vi "map Modbus channels.vi"(8 "error in":errorcluster, 10 "mapping":T1, 11 "Modbus Slave configuration in":refnum<class "Modbus Module configuration.lvclass">) -> (0 "error out":errorcluster, 3 "Modbus Slave configuration out":refnum<class "Modbus Module configuration.lvclass">)   [LabVIEW 2013, in "Modbus Module configuration.lvclass"]
uses:
  Modbus Module configuration.lvclass
  modbus mapping behavior.ctl
  Modbus Module configuration.lvclass/Modbus Module configuration.ctl
  <vilib>/NI/Tag Bus Module Framework/channel/channel classification.ctl
  module channel/data bank type.ctl
  <vilib>/NI/Tag Bus Module Framework/channel/TBM channel.lvclass/TBM channel.ctl
  module channel/Modbus Module Channel.lvclass/Modbus Module Channel.ctl
  <vilib>/NI/Tag Bus Module Framework/channel/Read channel classification.vi
  module channel/Read modbus type.vi
  module channel/Modbus Module Channel.lvclass
  <vilib>/NI/Tag Bus Module Framework/channel/TBM channel.lvclass
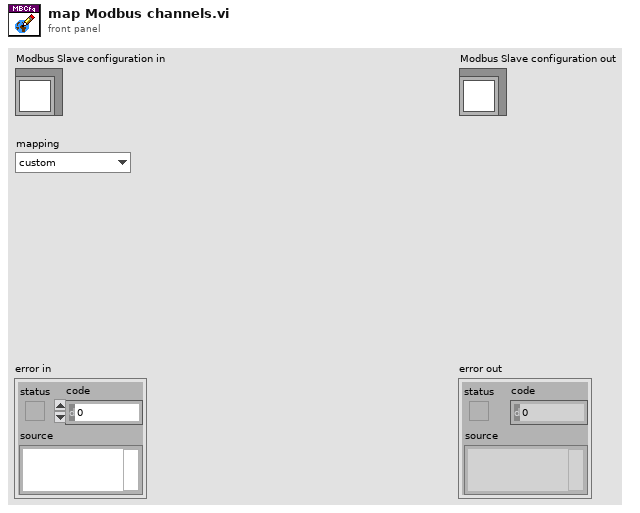
[diagram p1: front panel]
types:
  T1 = typedef "Modbus Module configuration.lvclass/modbus mapping behavior.ctl" = enum16{"custom", "optimized"}
  T2 = cluster{"starting address":u16, "subindex (bool)":i32}
  T3 = typedef "Modbus Module Channel.lvclass/data bank type.ctl" = enum16{"coils", "discrete inputs", "input registers", "holding registers"}
  T4 = typedef "TBM channel.lvclass/channel classification.ctl" = enum16{"input data", "output data", "processing parameter", "processing result"}
  T5 = cluster{"starting address":u16, "subindex (bool)":i32}[]
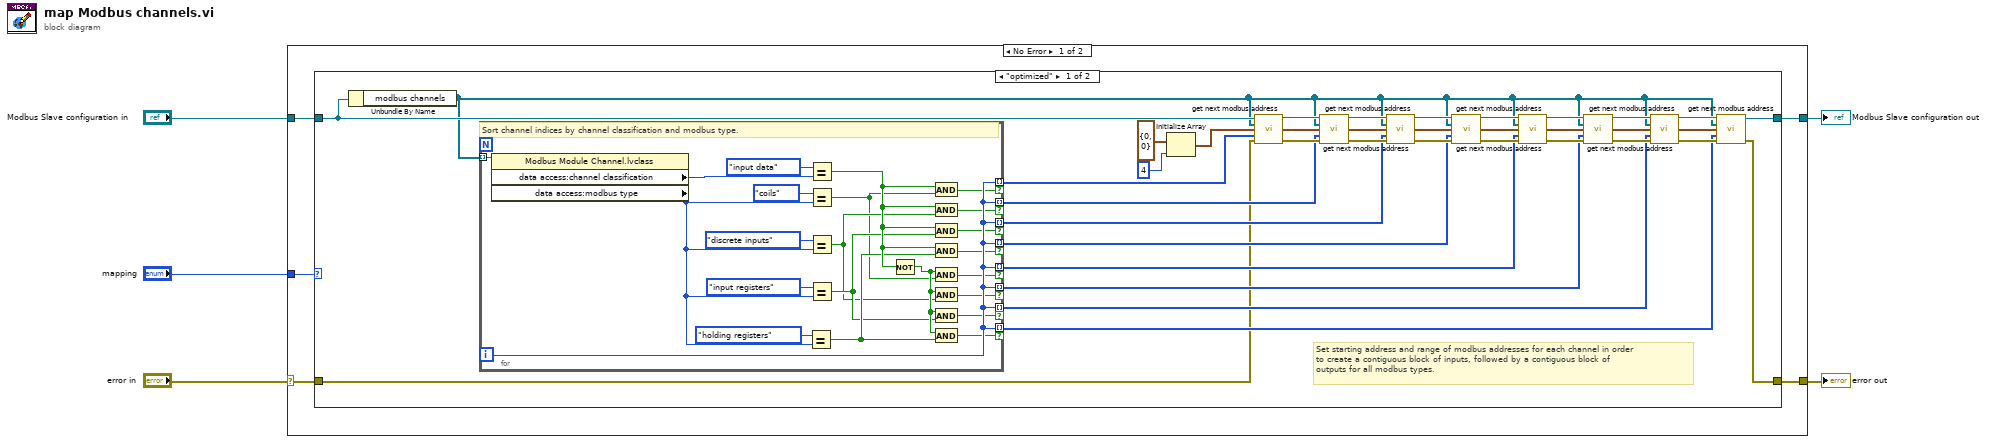
[diagram p0: block diagram]
diagram:
  n1 = case shown="No Error" "error in" {
    selector: "error in" -> [w10 w74]
    tunnel: [w7 w74] -> w4
    tunnel: [w8 w73] -> w2
    tunnel: "Modbus Slave configuration in" -> [w9 w73]
    tunnel: "mapping" -> [w6 _]
    frame No Error {
      n2 = case shown="\"optimized\"" w6 {
        tunnel: w10 -> [w12 w71]
        tunnel: w9 -> [w44 w72]
        tunnel: [w35 w72] -> w8
        tunnel: [w27 w71] -> w7
        frame "optimized" {
          # "Set starting address and range of modbus addresses for each channel in order\nto create a contiguous block of inputs, followed by a contiguous block of\noutputs for all modbus types."
          n3 = Unbundle By Name(w44) -> ("modbus channels"=w11:refnum<class "Modbus Module Channel.lvclass">[])
          n4 = for {
            tunnel: [w70] -> w43 mode=indexing if=w62
            tunnel: [w70] -> w19 mode=indexing if=w61
            tunnel: [w70] -> w18 mode=indexing if=w60
            tunnel: [w70] -> w17 mode=indexing if=w59
            tunnel: [w70] -> w15 mode=indexing if=w56
            tunnel: [w70] -> w14 mode=indexing if=w55
            tunnel: [w70] -> w13 mode=indexing if=w54
            tunnel: [w70] -> w16 mode=indexing if=w57
            tunnel: w11 -> [w48] mode=indexing
            i -> [w70]
            # "Sort channel indices by channel classification and modbus type."
            n5 = property class="Modbus Module Channel.lvclass"(reference=w48) -> ("data access:channel classification"=w69:T4, "data access:modbus type"=w63:T3)  [unwired: 1 in, 2 out]
            n6 = Equal?(x=data_bank_type."holding registers", y=w63) -> (x = y?=w52:bool)
            n7 = Equal?(x=channel_classification."input data", y=w69) -> (x = y?=w58:bool)
            n8 = Equal?(x=data_bank_type."coils", y=w63) -> (x = y?=w49:bool)
            n9 = Equal?(x=data_bank_type."discrete inputs", y=w63) -> (x = y?=w50:bool)
            n10 = Equal?(x=data_bank_type."input registers", y=w63) -> (x = y?=w51:bool)
            n11 = Not(x=w58) -> (.not. x?=w53:bool)
            n12 = And(x=w58, y=w49) -> (x .and. y?=w62:bool)
            n13 = And(x=w58, y=w50) -> (x .and. y?=w61:bool)
            n14 = And(x=w58, y=w51) -> (x .and. y?=w60:bool)
            n15 = And(x=w58, y=w52) -> (x .and. y?=w59:bool)
            n16 = And(x=w53, y=w49) -> (x .and. y?=w57:bool)
            n17 = And(x=w53, y=w50) -> (x .and. y?=w56:bool)
            n18 = And(x=w53, y=w51) -> (x .and. y?=w55:bool)
            n19 = And(x=w53, y=w52) -> (x .and. y?=w54:bool)
          }
          n20 = Initialize Array(T2 {"starting address"=0, "subindex (bool)"=0} ("next open address"), 4 ("dimension size")) -> (w45:T5)
          n21 = call "get next modbus address.vi"("Modbus Slave configuration in"=w44, "modbus channels"=w11, "modbus address"=w45, "channel indices"=w43, "error in"=w12) -> ("Modbus Slave configuration out"=w42:refnum<class "Modbus Module configuration.lvclass">, "modbus address out"=w26:T5, "error out"=w34:errorcluster)  [unwired: 8 in]
          n22 = call "get next modbus address.vi"("Modbus Slave configuration in"=w42, "modbus channels"=w11, "modbus address"=w26, "channel indices"=w19, "error in"=w34) -> ("Modbus Slave configuration out"=w41:refnum<class "Modbus Module configuration.lvclass">, "modbus address out"=w25:T5, "error out"=w33:errorcluster)  [unwired: 8 in]
          n23 = call "get next modbus address.vi"("Modbus Slave configuration in"=w41, "modbus channels"=w11, "modbus address"=w25, "channel indices"=w18, "error in"=w33) -> ("Modbus Slave configuration out"=w40:refnum<class "Modbus Module configuration.lvclass">, "modbus address out"=w24:T5, "error out"=w32:errorcluster)  [unwired: 8 in]
          n24 = call "get next modbus address.vi"("Modbus Slave configuration in"=w40, "modbus channels"=w11, "modbus address"=w24, "channel indices"=w17, "error in"=w32) -> ("Modbus Slave configuration out"=w39:refnum<class "Modbus Module configuration.lvclass">, "modbus address out"=w23:T5, "error out"=w31:errorcluster)  [unwired: 8 in]
          n25 = call "get next modbus address.vi"("Modbus Slave configuration in"=w39, "modbus channels"=w11, "modbus address"=w23, "channel indices"=w16, "error in"=w31) -> ("Modbus Slave configuration out"=w38:refnum<class "Modbus Module configuration.lvclass">, "modbus address out"=w22:T5, "error out"=w30:errorcluster)  [unwired: 8 in]
          n26 = call "get next modbus address.vi"("Modbus Slave configuration in"=w38, "modbus channels"=w11, "modbus address"=w22, "channel indices"=w15, "error in"=w30) -> ("Modbus Slave configuration out"=w37:refnum<class "Modbus Module configuration.lvclass">, "modbus address out"=w21:T5, "error out"=w29:errorcluster)  [unwired: 8 in]
          n27 = call "get next modbus address.vi"("Modbus Slave configuration in"=w37, "modbus channels"=w11, "modbus address"=w21, "channel indices"=w14, "error in"=w29) -> ("Modbus Slave configuration out"=w36:refnum<class "Modbus Module configuration.lvclass">, "modbus address out"=w20:T5, "error out"=w28:errorcluster)  [unwired: 8 in]
          n28 = call "get next modbus address.vi"("Modbus Slave configuration in"=w36, "modbus channels"=w11, "modbus address"=w20, "channel indices"=w13, "error in"=w28) -> ("Modbus Slave configuration out"=w35:refnum<class "Modbus Module configuration.lvclass">, "error out"=w27:errorcluster)  [unwired: 8 in, 1 out]
        }
        frame "custom", Default {
          # "A custom mapping is user-defined, \nso the configuration is left\nunchanged."
        }
      }
    }
    frame Error {
    }
  }
  "error out" <- w4
  "Modbus Slave configuration out" <- w2
